vi "Measure Output.vi"(8 "error in":errorcluster, 11 "69X_79X in":refnum<class "6972A.lvclass">) -> (0 "error out":errorcluster, 1 "Current":dbl[](array[numeric]), 2 "Voltage":dbl[](array[numeric]), 3 "69X_79X out":refnum<class "6972A.lvclass">)   [LabVIEW 2019, in "6972A.lvlib" / "6972A.lvclass"]
uses:
  Library/6972A.lvclass
  Library/6972A.lvclass/6972A.ctl
  <instrlib>/Agilent N6900 N7900 Series/Agilent N6900 N7900 Series.lvlib
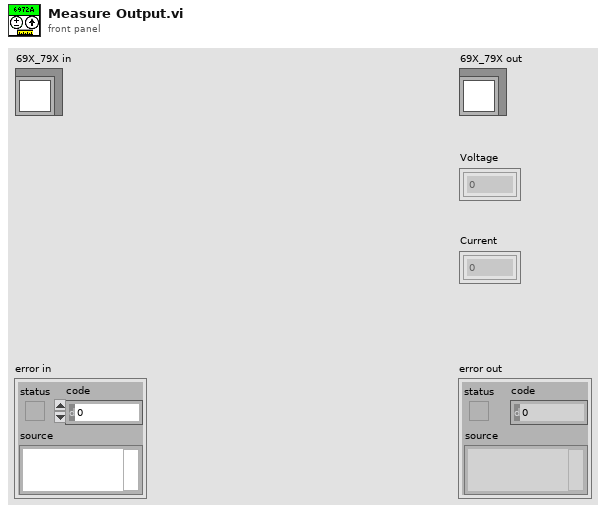
[diagram p1: front panel]
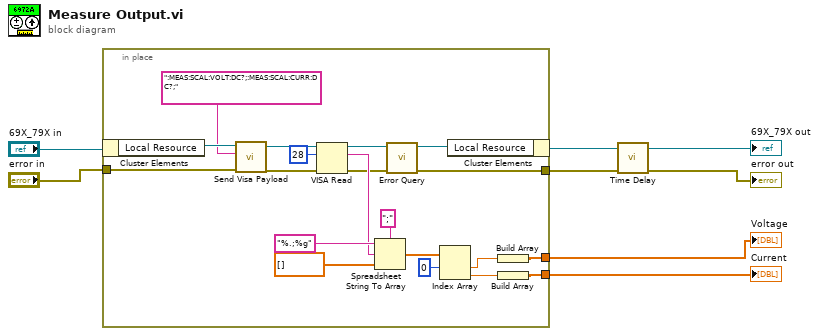
[diagram p0: block diagram]
diagram:
  n1 = in-place {
    in-place-border: "error in" -> [w25]
    in-place-border: [w8] -> w4
    in-place-border: [w13] -> w3
    in-place-border: [w12] -> w2
    n2 = in-place-cluster #1("69X_79X in") -> ("Local Resource"=w27:refnum<visa-resource-name>)
    n3 = call "Send Visa Payload.vi"("error in"=w25, "Command"=":MEAS:SCAL:VOLT:DC?;:MEAS:SCAL:CURR:DC?;", "Local Resource in"=w27) -> ("error out"=w24:errorcluster, "Local Resource out"=w26:refnum<visa-resource-name>)  [unwired: 7 in]
    n4 = VISA Read(VISA resource name=w26, byte count=u32 28, error in (no error)=w24) -> (VISA resource name out=w11:refnum<visa-resource-name>, read buffer=w14:string, error out=w10:errorcluster)  [unwired: 1 out]
    n5 = Spreadsheet String To Array(delimiter (Tab)=";", format string="%.;%g", spreadsheet string=w14, array type (2D Dbl)=dbl[] []) -> (array=w18:dbl[])
    n6 = call <instrlib>:"Error Query.vi"("error in (no error)"=w10, "VISA resource name"=w11) -> ("error out"=w8:errorcluster, "VISA resource name out"=w9:refnum<visa-resource-name>)  [unwired: 6 in, 2 out]
    n7 = Index Array(array=w18, index #1=0 ("index")) -> (element #1=w20:dbl, element #2=w21:dbl)  [unwired: 1 in]
    n8 = in-place-cluster #1("Local Resource"=w9) -> (→"69X_79X out":refnum<class "6972A.lvclass">)
    n9 = Build Array(w20) -> (w13:dbl[])
    n10 = Build Array(w21) -> (w12:dbl[])
  }
  "Current" <- w2
  "Voltage" <- w3
  n11 = call "Time Delay"("error in (no error)"=w4) -> ("error out"=→"error out":errorcluster)  [unwired: 10 in]
